vi "2 SailControlFunction.vi"() -> (2 "Sail Position":T2)   [LabVIEW 2011]
doc: "Sets the desired sail position based on the apparent wind direction.\nWe used to set sail from a lookup table, but now we use either a trigonometric or a linear function."
uses:
  2 Globals/2 Global.vi
  2 Globals/2 TuningConstants.vi
  2 Typedefs/sail setpt.ctl
  0x2-OCU-Think Comm/0x2 Typedefs/Sail Setting Tuning.ctl
panel:
  out "Sail Setting Options":T1={"Linear\nMode"=FALSE, "Sails Full In Point"=45.0, "Sails Full Out Point"=180.0} {"Sails Full Out Point" step=0.1; "Sails Full In Point" step=0.1}
  # "135"
  # "180"
  # "315"
  # "360"
  # "180"
  # "135"
  # "315"
  # "360"
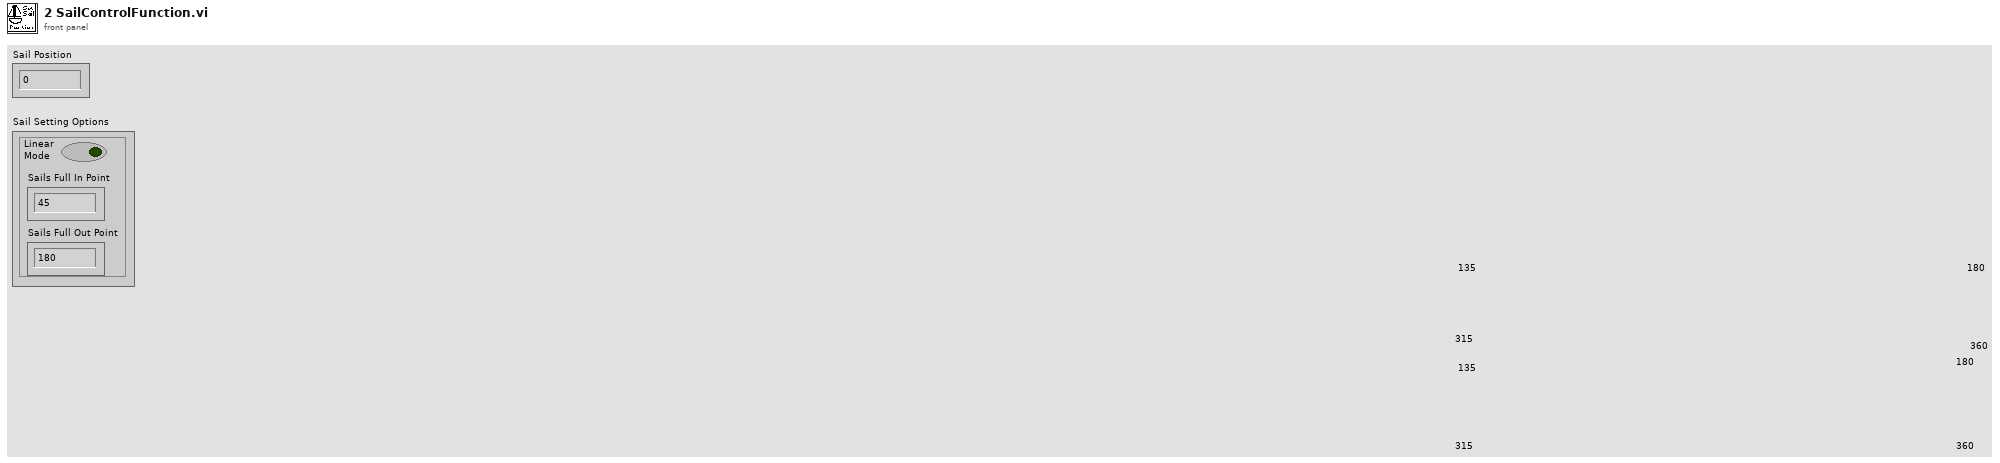
[diagram p1: front panel]
types:
  T1 = typedef "Sail Setting Tuning.ctl" = cluster{"Linear\nMode":bool, "Sails Full In Point":dbl, "Sails Full Out Point":dbl}
  T2 = typedef "sail setpt.ctl" = dbl
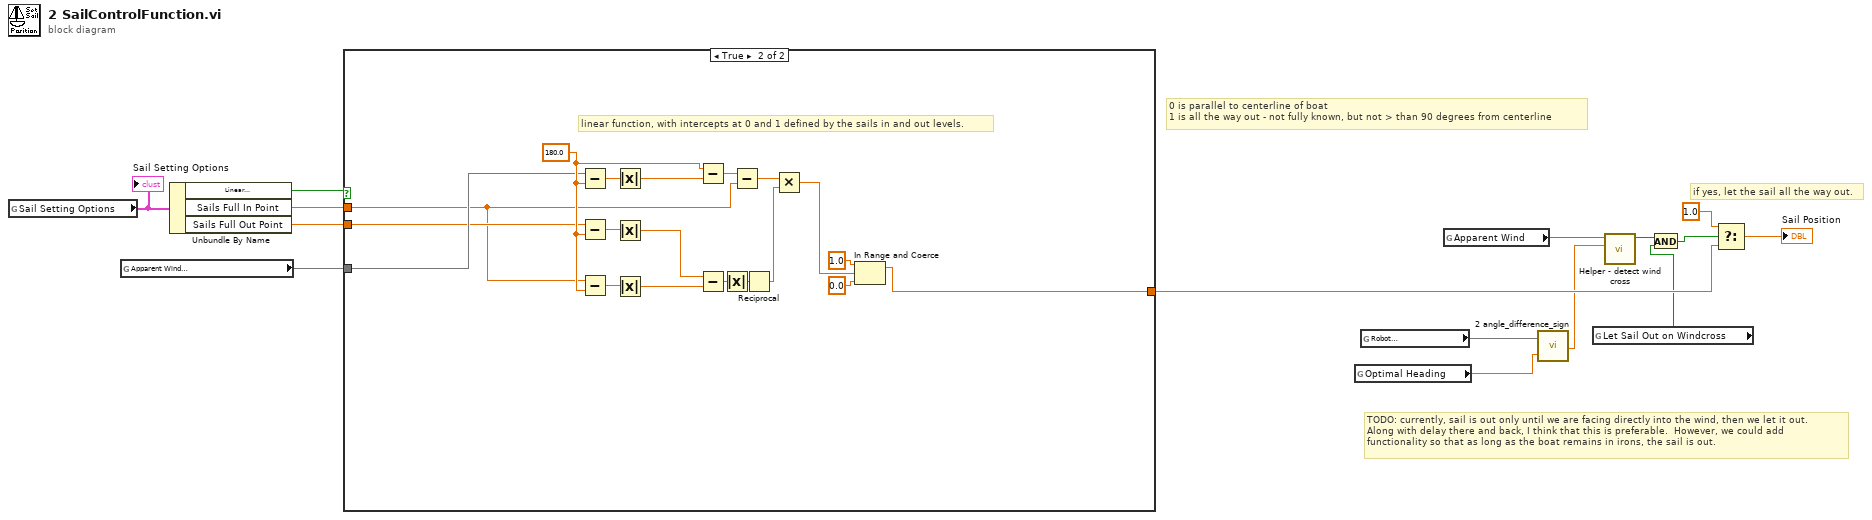
[diagram p0: block diagram]
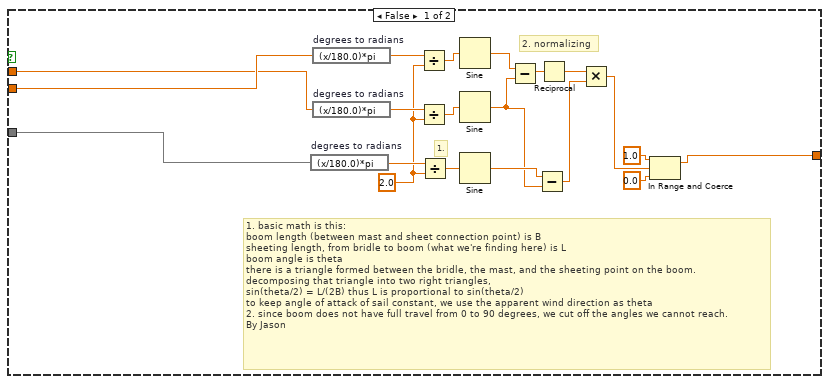
[diagram p2: hidden frame]
diagram:
  # "TODO: currently, sail is out only until we are facing directly into the wind, then we let it out.\nAlong with delay there and back, I think that this is preferable.  However, we could add \nfunctionality so that as long as the boat remains in irons, the sail is out."
  # "if yes, let the sail all the way out."
  # "0 is parallel to centerline of boat\n1 is all the way out - not fully known, but not > than 90 degrees from centerline"
  n1 = global read "2 TuningConstants.vi" "Sail Setting Options"() -> (w8:T1)
  "Sail Setting Options" <- w8
  n2 = global read "2 Global.vi" "Apparent Wind\nDirection (º)"() -> (w1)
  n3 = Unbundle By Name(w8) -> ("Linear\nMode"=w7:bool, "Sails Full In Point"=w5:dbl, "Sails Full Out Point"=w6:dbl)
  n4 = case shown="True" w7 {
    tunnel: [w20 w38] -> w13
    tunnel: w1 -> [w19 w39]
    tunnel: w6 -> [w18 w37]
    tunnel: w5 -> [w17 w36]
    frame False {
      w21 = 2.0 ("x")
      # "2. normalizing"
      # "1."
      # "1. basic math is this: \nboom length (between mast and sheet connection point) is B\nsheeting length, from bridle to boom (what we're finding here) is L\nboom angle is theta\nthere is a triangle formed between the bridle, the mast, and the sheeting point on the boom.\ndecomposing that triangle into two right triangles,\nsin(theta/2) = L/(2B) thus L is proportional to sin(theta/2)\nto keep angle of attack of sail constant, we use the apparent wind direction as theta\n2. since boom does not have full travel from 0 to 90 degrees, we cut off the angles we cannot reach.\nBy Jason"
      n5 = expression code="(x/180.0)*pi" "degrees to radians"(w19) -> (w35:dbl)
      n6 = expression code="(x/180.0)*pi" "degrees to radians"(w18) -> (w27:dbl)
      n7 = expression code="(x/180.0)*pi" "degrees to radians"(w17) -> (w30:dbl)
      n8 = Divide(x=w27, y=w21) -> (x/y=w28:dbl)
      n9 = Divide(x=w30, y=w21) -> (x/y=w29:dbl)
      n10 = Divide(x=w35, y=w21) -> (x/y=w34:dbl)
      n11 = Sine(x=w28) -> (sin(x)=w26:dbl)
      n12 = Sine(x=w29) -> (sin(x)=w16:dbl)
      n13 = Sine(x=w34) -> (sin(x)=w31:dbl)
      n14 = Subtract(x=w26, y=w16) -> (x-y=w25:dbl)
      n15 = Subtract(x=w31, y=w16) -> (x-y=w23:dbl)
      n16 = Reciprocal(x=w25) -> (1/x=w24:dbl)
      n17 = Multiply(x=w24, y=w23) -> (x*y=w22:dbl)
      n18 = In Range and Coerce(upper limit=1.0, x=w22, lower limit=0.0 ("upper limit")) -> (coerced(x)=w20:dbl)  [unwired: 1 out]
    }
    frame True {
      w44 = 180.0 ("upper limit")
      # "linear function, with intercepts at 0 and 1 defined by the sails in and out levels."
      n19 = Subtract(x=w39, y=w44) -> (x-y=w52:dbl)
      n20 = Subtract(x=w37, y=w44) -> (x-y=w51:dbl)
      n21 = Subtract(x=w36, y=w44) -> (x-y=w50:dbl)
      n22 = Absolute Value(x=w52) -> (abs(x)=w48:dbl)
      n23 = Absolute Value(x=w51) -> (abs(x)=w40:dbl)
      n24 = Absolute Value(x=w50) -> (abs(x)=w41:dbl)
      n25 = Subtract(x=w44, y=w48) -> (x-y=w43:dbl)
      n26 = Subtract(x=w40, y=w41) -> (x-y=w49:dbl)
      n27 = Absolute Value(x=w49) -> (abs(x)=w45:dbl)
      n28 = Subtract(x=w43, y=w36) -> (x-y=w42:dbl)
      n29 = Reciprocal(x=w45) -> (1/x=w47:dbl)
      n30 = Multiply(x=w42, y=w47) -> (x*y=w46:dbl)
      n31 = In Range and Coerce(upper limit=1.0, x=w46, lower limit=0.0 ("upper limit")) -> (coerced(x)=w38:dbl)  [unwired: 1 out]
    }
  }
  n32 = global read "2 Global.vi" "Optimal Heading"() -> (w15:dbl)
  n33 = global read "2 Global.vi" "Robot\nHeading"() -> (w9)
  n34 = global read "2 Global.vi" "Apparent Wind"() -> (w3)
  n35 = call "2 angle_difference_sign.vi"("Angle 2"=w15, "Angle 1"=w9) -> ("Difference"=w2:dbl)
  n36 = global read "2 Global.vi" "Let Sail Out on Windcross"() -> (w10:bool)
  n37 = call "Helper - detect wind cross.vi"("Heading Change"=w2, "Apparent Wind"=w3) -> ("Crossing Wind?"=w4:bool)  [unwired: 9 in]
  n38 = And(x=w4, y=w10) -> (x .and. y?=w11:bool)
  n39 = Select(t=1.0 ("f"), s=w11, f=w13) -> (s? t:f=→"Sail Position":dbl)
